vi "Initialize.vi"(8 "error in (no error)":errorcluster, 11 "Sequencer State Machine in":refnum<class "Sequencer State Machine.lvclass">) -> (0 "error out":errorcluster, 3 "Sequencer State Machine out":refnum<class "Sequencer State Machine.lvclass">)   [LabVIEW 2018, in "Sequencer State Machine.lvclass"]
uses:
  Sequencer State Machine.lvclass
  Sequencer State.ctl
  Sequencer State Machine.lvclass/Sequencer State Machine.ctl
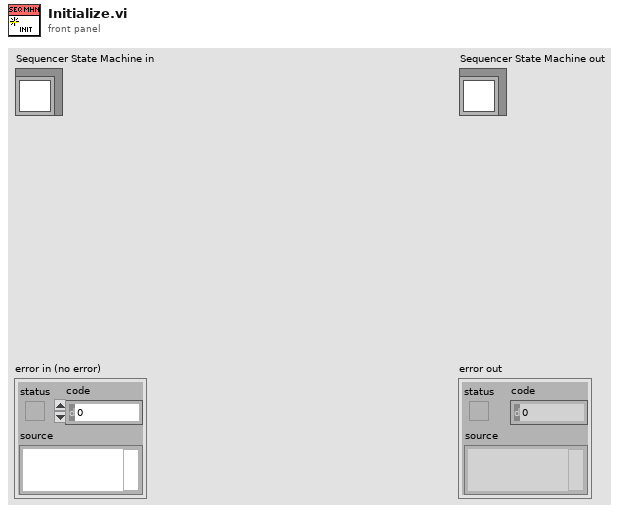
[diagram p1: front panel]
types:
  T1 = typedef "Sequencer State.ctl" = enum16{"Idle", "Starting", "Waiting for primary", "Waiting for secondary"}
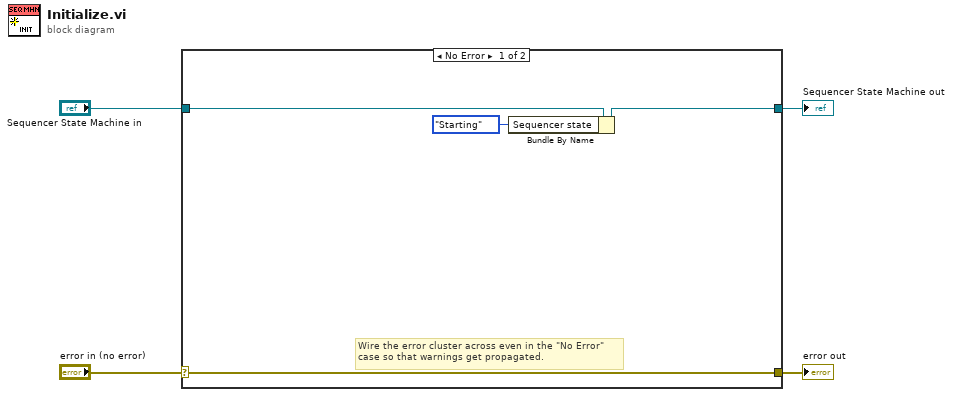
[diagram p0: block diagram]
diagram:
  n1 = case shown="No Error" "error in (no error)" {
    selector: "error in (no error)" -> [w7 w10]
    tunnel: [w7 w10] -> w3
    tunnel: [w6 w9] -> w1
    tunnel: "Sequencer State Machine in" -> [w8 w9]
    frame No Error {
      # "Wire the error cluster across even in the \"No Error\"\ncase so that warnings get propagated."
      n2 = Bundle By Name(cluster=w8, "Sequencer state"=Sequencer_State."Starting") -> (w6:refnum<class "Sequencer State Machine.lvclass">)
    }
    frame Error {
    }
  }
  "error out" <- w3
  "Sequencer State Machine out" <- w1
